vi "VNA_config_freq_sweep.vi"(4 "IF Bandwidth":dbl, 5 "Averaging":i32, 6 "Number of Points":i32, 7 "Output Power":dbl, 8 "error in (no error)":errorcluster, 9 "Stop Frequency":dbl, 10 "Start Frequency":dbl, 11 "Resource Name In":refnum<k15>) -> (0 "error out":errorcluster, 3 "Resource Name Out":refnum<k15>)   [LabVIEW 2017]
uses:
  <instrlib>/niVNA/niVNA.llb/niVNA Configure Frequency Start Stop.vi
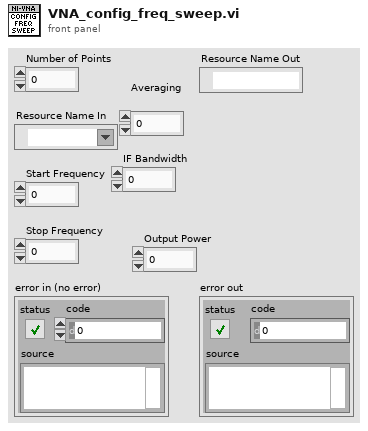
[diagram p1: front panel]
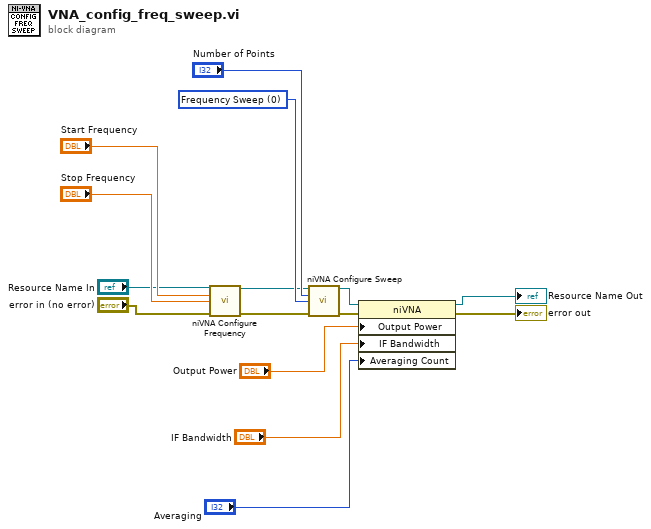
[diagram p0: block diagram]
diagram:
  w12 = 0 items=["Frequency Sweep", "Power Sweep"] ("sweep mode")
  n1 = call-poly <instrlib>:"niVNA Configure Frequency.vi"("instrument handle"="Resource Name In", "start frequency"="Start Frequency", "stop frequency"="Stop Frequency", "error in"="error in (no error)") -> ("instrument handle out"=w10:refnum<k15>, "error out"=w11:errorcluster)  [unwired: 10 in]
  n2 = call <instrlib>:"niVNA Configure Sweep.vi"("instrument handle"=w10, "number of points"="Number of Points", "sweep mode"=w12, "error in"=w11) -> ("instrument handle out"=w9:refnum<k15>, "error out"=w8:errorcluster)  [unwired: 10 in]
  n3 = property class="niVNA"(reference=w9, error in=w8, "Output Power"="Output Power", "IF Bandwidth"="IF Bandwidth", "Averaging Count"="Averaging") -> (reference out=→"Resource Name Out":refnum<k15>, error out=→"error out":errorcluster)
